vi "POP send RETR.vi"(3 "error in":errorcluster, 4 "MSG number":i32=1, 5 "connection ID in":refnum<k5>) -> (0 "error out":errorcluster, 1 "RETR response":string="\r\n", 2 "connection ID out":refnum<k5>)   [LabVIEW 2012]
doc: "This low-level POP VI sends the \"RETR\" command to a mail server, instructing it to send the contents of the specified message back to the client. The message number argument can range from 1 to N, assuming there are N messages stored on the server."
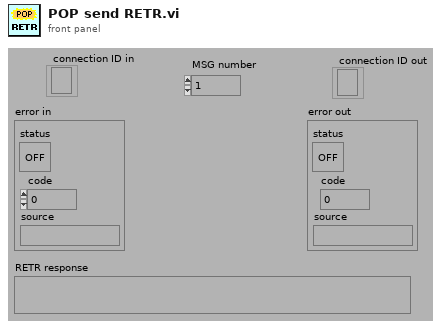
[diagram p1: front panel]
types:
  T1 = enum16{"Standard", "Buffered", "CRLF", "Immediate"}
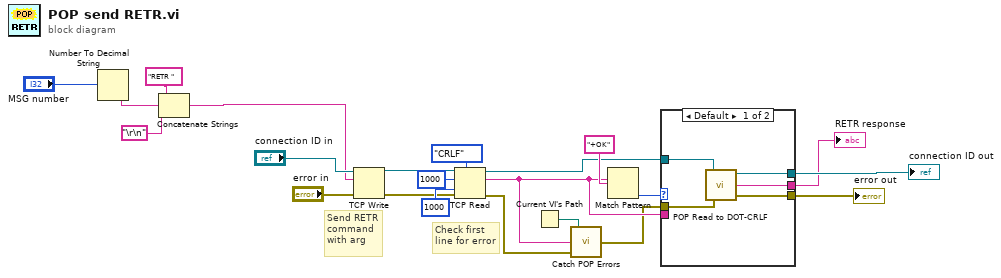
[diagram p0: block diagram]
diagram:
  # "Check first\nline for error"
  # "Send RETR\ncommand\nwith arg"
  n1 = Number To Decimal String(number="MSG number") -> (decimal integer string=w13:string)  [unwired: 1 in]
  n2 = Concatenate Strings("RETR ", w13, "\r\n") -> (w16:string)
  n3 = TCP Write(connection ID="connection ID in", data in=w16, error in (no error)="error in") -> (connection ID out=w9:refnum<k5>, error out=w8:errorcluster)  [unwired: 1 in, 1 out]
  n4 = TCP Read(connection ID=w9, bytes to read=1000, error in (no error)=w8, 7:T1."CRLF" ("mode (standard)"), 9:1000 ("timeout ms (25000)")) -> (connection ID out=w5:refnum<k5>, data out=w3:string, error out=w2:errorcluster)
  n5 = Current VI's Path() -> (path=w4:path)
  n6 = call "Catch POP Errors.vi"("error in"=w2, "POP server response"=w3, "Caller Path"=w4) -> ("error out"=w1:errorcluster)
  n7 = Match Pattern(string=w3, regular expression="+OK") -> (offset past match=w6:i32)  [unwired: 1 in, 3 out]
  n8 = case shown="Default" w6 {
    tunnel: [w27 w28] -> w20
    tunnel: [w26 w29] -> w19
    tunnel: [w25 w30] -> w18
    tunnel: w3 -> [_ w30]
    tunnel: w1 -> [w24 w29]
    tunnel: w5 -> [w23 w28]
    frame Default {
      n9 = call "POP Read to DOT-CRLF.vi"("error in"=w24, "connection ID in"=w23) -> ("error out"=w26:errorcluster, "LIST response"=w25:string, "connection ID out"=w27:refnum<k5>)  [unwired: 1 in]
    }
    frame -1 {
    }
  }
  "error out" <- w19
  "RETR response" <- w18
  "connection ID out" <- w20
